vi "HS_DAQ_RealTime.vi"() -> ()   [LabVIEW 2020]
uses:
  Program Files (x86)/National Instruments/LabVIEW 2020/examples/CompactRIO/Shared/cRIO Convert Thermocouple Readings.llb/Thermocouple Type.ctl
  <vilib>/FPGAPlugInAG/cRIO-9064/niLvFpga_Open_cRIO-9064.vi
  <vilib>/rvi/interface/common/dynamic/niFpgaDynamicAddResources.vi
  <vilib>/Utility/error.llb/Error Cluster From Error Code.vi
  <vilib>/rvi/errors/niLvFpgaAdjustHostInterfaceError.vi
  Program Files (x86)/National Instruments/LabVIEW 2020/examples/CompactRIO/Module Specific/NI 9214/NI 9214 Support Files.llb/NI 9214 Convert to Temperature (Calibrated).vi
  <vilib>/FPGAPlugInAG/Dynamic/niLvFpga_Close_Dynamic.vi
  <vilib>/rvi/interface/nirviOpenFPGA/nirviOpenFPGA.xnode
  FPGA Bitfiles/hsdaq_FPGATarget_HSDAQFPGA_s3VrIaQjD7I.lvbitx
  HS_DAQ_FPGA.vi
  <vilib>/rvi/interface/nirviReadWriteControl/nirviReadWriteControl.xnode
  <vilib>/rvi/interface/nirviMethod/nirviMethod.xnode
  <vilib>/rvi/interface/nirviCloseFPGA/nirviCloseFPGA.xnode
  <vilib>/FPGAPlugInAG/Dynamic/niLvFpga_ReadFifo_Dynamic.vi
  <vilib>/rvi/errors/niLvFpgaMergeErrorWithErrorCode.vi
  <vilib>/rvi/interface/Simulation/niFpgaSimulationCallBeginRW.vi
  NiFpgaLv.dll
panel:
  out "Consumer loop time [us]":u32
  out "Producer loop time [us]":u32
  out "Thermocouple Temperature":dbl
  out "Queue in":dbl[][](array[numeric])
  out "Queue out":dbl[][](array[numeric])
  out "error out":errorcluster
  in  "Points per block read":u32=200
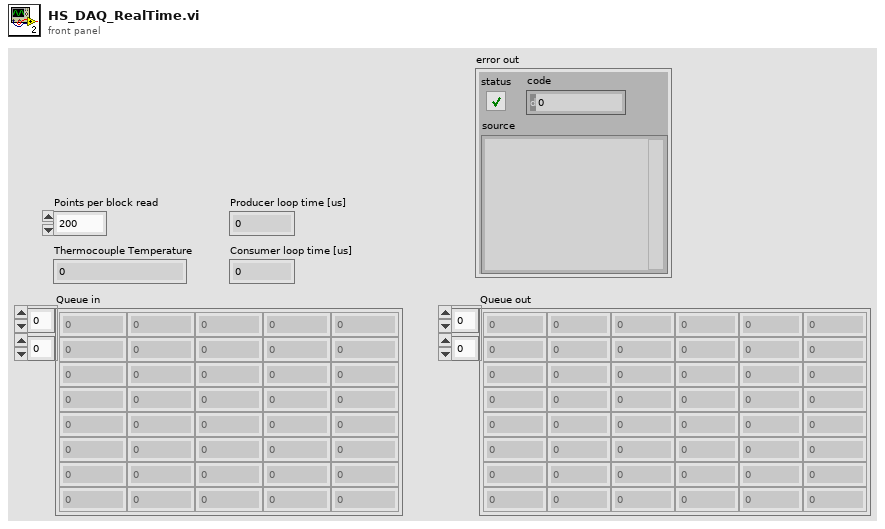
[diagram p1: front panel]
types:
  T1 = typedef "Thermocouple Type.ctl" = u16
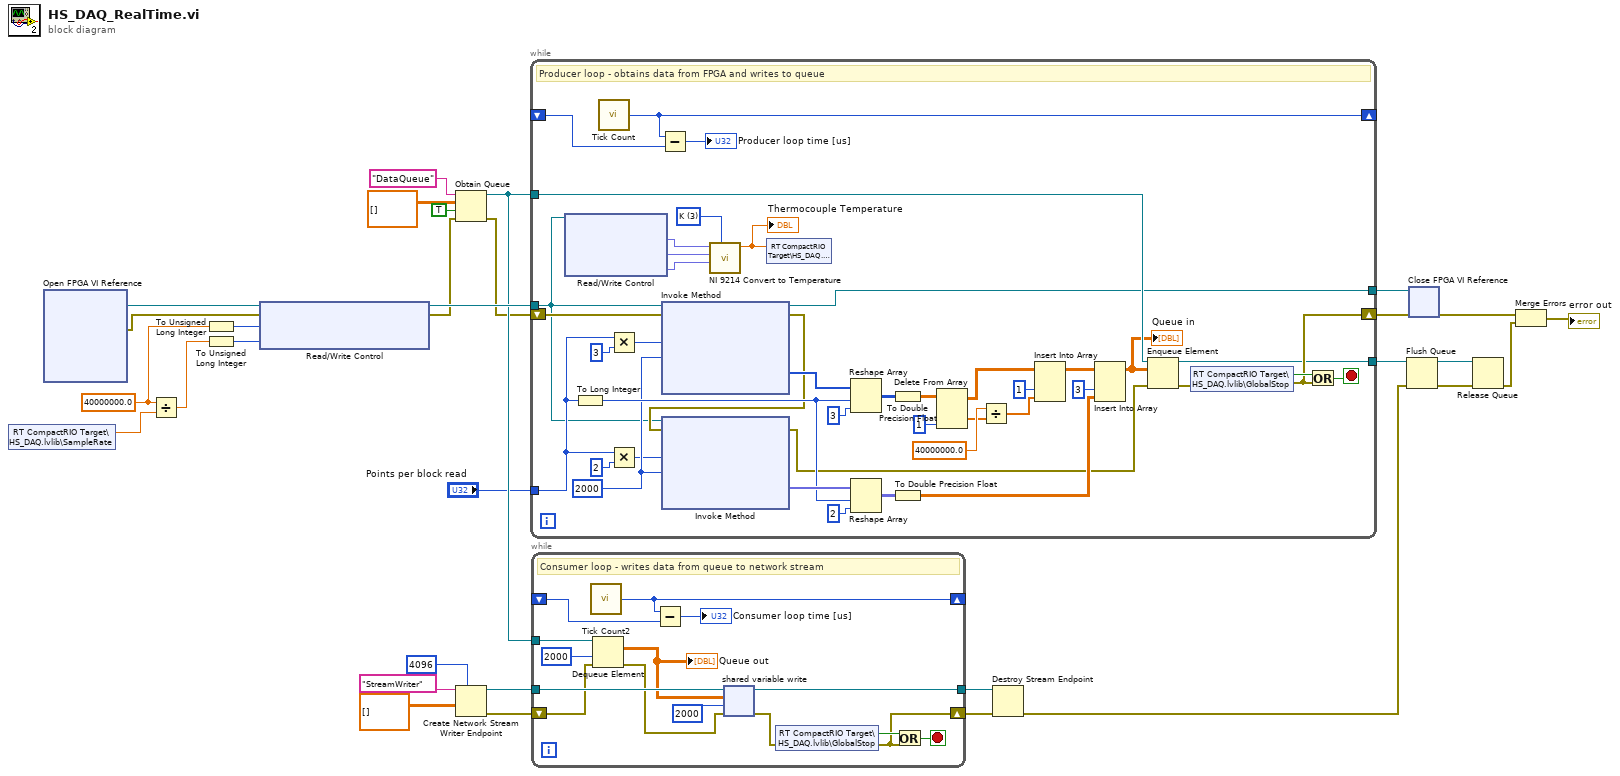
[diagram p0: block diagram]
diagram:
  w10 = 40000000.0 ("x")
  n1 = shared-variable "RT CompactRIO Target\\HS_DAQ.lvlib\\SampleRate"() -> (w30:dbl)  [unwired: 1 in, 1 out]
  n2 = xnode "Open FPGA VI Reference"() -> ("FPGA VI Reference Out"=w31:refnum<k20>, "error out"=w26:errorcluster)  [unwired: 2 in]
  n3 = Divide(x=w10, y=w30) -> (x/y=w9:dbl)
  n4 = To Unsigned Long Integer(number=w10) -> (unsigned 32bit integer=w15:u32)
  n5 = To Unsigned Long Integer(number=w9) -> (unsigned 32bit integer=w14:u32)
  n6 = xnode "Read/Write Control"("FPGA VI Reference In"=w31, "error in"=w26, "Temp sample period [ticks]"=w15, "Analog sample period [ticks]"=w14) -> ("FPGA VI Reference Out"=w29:refnum<k20>, "error out"=w8:errorcluster)
  n7 = Obtain Queue(name (unnamed)="DataQueue", element data type=dbl[][] [], create if not found? (T)=TRUE, error in (no error)=w8) -> (queue out=w25:refnum<queue>, error out=w7:errorcluster)  [unwired: 1 in, 1 out]
  n8 = Create Network Stream Writer Endpoint(7:4096 ("writer buffer size"), 9:dbl[][] [], 11:"StreamWriter" ("writer name")) -> (0:w20:errorcluster, 3:w22:refnum<k21>)  [unwired: 4 in]
  n9 = while {
    tunnel: w29 -> [w40]
    tunnel: w25 -> [w71]
    shift-right: [w50] -> w13
    shift-left: w7 -> [w70]
    tunnel: "Points per block read" -> [w55]
    tunnel: [w59] -> w12
    tunnel: [w49] -> w5
    shift-right: [w34] -> _
    shift-left: _ -> [w33]
    stop <- w51 stop-if-true
    w36 = T1 3 items=["B", "E", "J", "K", "R", "S", "T", "N"] ("ThermocoupleType")
    w61 = 2000 ("Timeout (ms)")
    # "Producer loop - obtains data from FPGA and writes to queue"
    n10 = xnode "Read/Write Control"("FPGA VI Reference In"=w40) -> ("TC0"=w39:fxp<+/-,24,-2>, "Mod3/CJC0"=w38:fxp<+/-,24,-2>, "Mod3/Autozero"=w37:fxp<+/-,24,-2>)  [unwired: 1 in, 2 out]
    n11 = To Long Integer(number=w55) -> (32bit integer=w66:i32)
    n12 = call "Tick Count"() -> ("Tick Count(uSec)"=w34:u32)
    n13 = Multiply(x=w55, y=u32 3) -> (x*y=w68:u32)
    n14 = Multiply(x=w55, y=u32 2) -> (x*y=w56:u32)
    n15 = Subtract(x=w34, y=w33) -> (x-y=→"Producer loop time [us]":u32)
    n16 = xnode "Invoke Method"("FPGA VI Reference In"=w40, "error in"=w70, "Number of Elements"=w68, "Timeout (ms)"=w61) -> ("FPGA VI Reference Out"=w59:refnum<k20>, "error out"=w60:errorcluster, "Data"=w73:u32[])  [unwired: 1 out]
    n17 = xnode "Invoke Method"("FPGA VI Reference In"=w40, "error in"=w60, "Number of Elements"=w56, "Timeout (ms)"=w61) -> ("error out"=w58:errorcluster, "Data"=w67:fxp<+/-,26,5>[])  [unwired: 2 out]
    n18 = call-poly "NI 9214 Convert to Temperature.vi"("ThermocoupleType"=w36, "AutoZero"=w37, "CJC"=w38, "TC Input"=w39) -> ("Thermocouple Temperature"=w35:dbl)  [unwired: 7 in]
    "Thermocouple Temperature" <- w35
    n19 = shared-variable "RT CompactRIO Target\\HS_DAQ.lvlib\\TC0"(w35) -> ()  [unwired: 1 in, 1 out]
    n20 = Reshape Array(w73, w66, 3 ("dimension size")) -> (w72:u32[][])
    n21 = Reshape Array(w67, w66, 2 ("dimension size")) -> (w64:fxp<+/-,26,5>[][])
    n22 = To Double Precision Float(number=w72) -> (double precision float=w47:dbl[][])
    n23 = To Double Precision Float(number=w64) -> (double precision float=w63:dbl[][])
    n24 = Delete From Array(array=w47, index (col)=1 ("disabled index (col)")) -> (deleted portion=w45:dbl[], array with subset deleted=w44:dbl[][])  [unwired: 2 in]
    n25 = Divide(x=40000000.0, y=w45) -> (x/y=w43:dbl[])
    n26 = Insert Into Array(array=w44, index (col)=1 ("disabled index (col)"), new element=w43) -> (w42:dbl[][])  [unwired: 1 in]
    n27 = Insert Into Array(array=w42, index (col)=3 ("disabled index (col)"), new element=w63) -> (w62:dbl[][])  [unwired: 1 in]
    "Queue in" <- w62
    n28 = Enqueue Element(queue=w71, element=w62, error in (no error)=w58) -> (queue out=w49:refnum<queue>, error out=w57:errorcluster)  [unwired: 1 in, 1 out]
    n29 = shared-variable "RT CompactRIO Target\\HS_DAQ.lvlib\\GlobalStop"(error in=w57) -> (w52:bool, error out=w50:errorcluster)
    n30 = Or(x=w52, y=w50) -> (x .or. y?=w51:bool)
  }
  n31 = while {
    tunnel: w25 -> [w89]
    tunnel: w22 -> [w88]
    tunnel: [w86] -> w2
    shift-right: [w78] -> w1
    shift-left: w20 -> [w84]
    shift-right: [w77] -> _
    shift-left: _ -> [w76]
    stop <- w80 stop-if-true
    # "Consumer loop - writes data from queue to network stream"
    n32 = call "Tick Count2"() -> ("Tick Count(uSec)"=w77:u32)
    n33 = Dequeue Element(queue=w89, timeout in ms (-1)=2000, error in (no error)=w84) -> (element=w87:dbl[][], error out=w85:errorcluster)  [unwired: 2 out]
    "Queue out" <- w87
    n34 = Subtract(x=w77, y=w76) -> (x-y=→"Consumer loop time [us]":u32)
    n35 = shared-variable-write(w88, w85, w87, 2000 ("timeout ms (-1)")) -> (w86:refnum<k21>, w79:errorcluster)  [unwired: 1 out]
    n36 = shared-variable "RT CompactRIO Target\\HS_DAQ.lvlib\\GlobalStop"(error in=w79) -> (w81:bool, error out=w78:errorcluster)
    n37 = Or(x=w81, y=w78) -> (x .or. y?=w80:bool)
  }
  n38 = Destroy Stream Endpoint(8:w1, 11:w2) -> (0:w4:errorcluster)
  n39 = Flush Queue(queue=w5, error in (no error)=w4) -> (queue out=w21:refnum<queue>, error out=w19:errorcluster)  [unwired: 1 out]
  n40 = xnode "Close FPGA VI Reference"("FPGA VI Reference In"=w12, "error in"=w13) -> ("error out"=w11:errorcluster)
  n41 = Release Queue(queue=w21, error in (no error)=w19) -> (error out=w3:errorcluster)  [unwired: 1 in, 2 out]
  n42 = Merge Errors(w11, w3) -> (→"error out":errorcluster)
